vi "Panel by Name.vi"(7 "Panel Type (Base)":refnum<class "Panel.lvclass">, 8 "error in (no error)":errorcluster, 10 "Name":string, 11 "PanelManager in":refnum<class "PanelManager.lvclass">) -> (0 "error out":errorcluster, 2 "Panel":refnum<class "Panel.lvclass">, 3 "PanelManager out":refnum<class "PanelManager.lvclass">)   [LabVIEW 2018, in "OOPanel.lvlib" / "PanelManager.lvclass"]
uses:
  PanelManager.lvclass
  Panel/Panel.lvclass
  PanelManager.lvclass/PanelManager.ctl
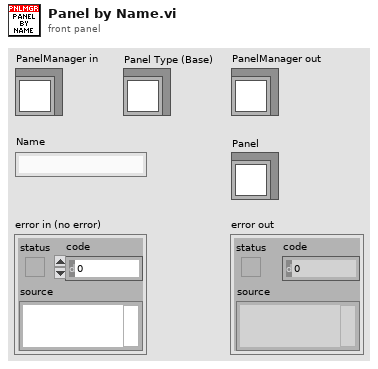
[diagram p1: front panel]
types:
  T1 = typedef "OOPanel.lvlib/PanelManager.lvclass/Ref Data.ctl" = cluster{"Panels":T2, "Subpanel Map":T3}
  T2 = typedef "OOPanel.lvlib/PanelManager.lvclass/Panels.ctl" = cluster{"Names":string[], "Instances":refnum<class "Panel.lvclass">[]}
  T3 = typedef "OOPanel.lvlib/PanelManager.lvclass/SubPanel Map.ctl" = cluster{"SubPanels":refnum<vi>[], "Panels":refnum<class "Panel.lvclass">[]}
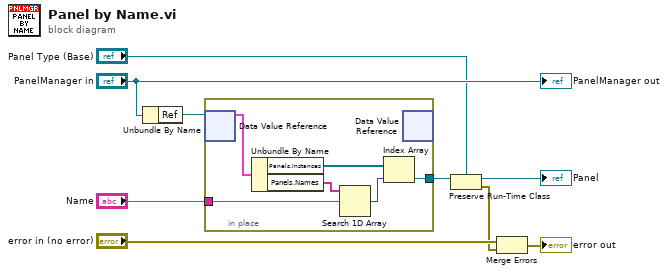
[diagram p0: block diagram]
diagram:
  n1 = Unbundle By Name("PanelManager in") -> ("Ref"=w7:refnum<data-value>)
  n2 = in-place {
    in-place-border: [w11] -> w6
    in-place-border: "Name" -> [w10]
    n3 = in-place-dvr #1(w7) -> (w15:T1)  [unwired: 1 out]
    n4 = Unbundle By Name(w15) -> ("Panels.Instances"=w14:refnum<class "Panel.lvclass">[], "Panels.Names"=w13:string[])
    n5 = Search 1D Array(1D array=w13, element=w10) -> (index of element=w12:i32)  [unwired: 1 in]
    n6 = Index Array(array=w14, index=w12) -> (element=w11:refnum<class "Panel.lvclass">)
    n7 = in-place-dvr #1() -> ()  [unwired: 1 in, 2 out]
  }
  n8 = Preserve Run-Time Class(object in=w6, 2:"Panel Type (Base)") -> (object out=→"Panel":refnum<class "Panel.lvclass">, error out=w1:errorcluster)  [unwired: 1 in]
  n9 = Merge Errors("error in (no error)", w1) -> (→"error out":errorcluster)
  "PanelManager out" <- "PanelManager in"
